vi "Build Update.vi"(8 "error in (no error)":errorcluster, 9 "tableName":string, 10 "DynamicParameters in":refnum<class "DynamicParameters.lvclass">, 11 "KDBConnection in":refnum<class "DBC.lvclass">) -> (0 "error out":errorcluster, 2 "Query":string, 3 "KDBConnection out":refnum<class "DBC.lvclass">)   [LabVIEW 2020, in "ORM_DBC_Kdb.lvlib" / "DBC.lvclass"]
uses:
  DBC.lvclass
  C:/Program Files/National Instruments/LabVIEW 2020/vi.lib/Viviota/shared/ORM.lvlibp/ORM/DbConnection/DbConnection.lvclass
  <vilib>/Viviota/shared/ORM.lvlibp/ORM/DynamicParameters/DynamicParameters.lvclass
  <vilib>/Viviota/shared/ORM.lvlibp/ORM/DbConnection/Read ColumnNameEqualsValueFormat.vi
  <vilib>/Viviota/shared/ORM.lvlibp/ORM/DbConnection/Write ExecuteScalar.vi
  <vilib>/Viviota/shared/ORM.lvlibp/ORM/DynamicParameters/Read FieldNames.vi
  <vilib>/Viviota/shared/ORM.lvlibp/ORM/DynamicParameters/Read ParameterNames.vi
  <vilib>/Viviota/shared/ORM.lvlibp/ORM/DynamicParameters/Read KeyProperties.vi
  <vilib>/Viviota/shared/ORM.lvlibp/ORM/DynamicParameters/Read AutoKey.vi
  <vilib>/Viviota/shared/ORM.lvlibp/ORM/DynamicParameters/Read ParameterOptions.vi
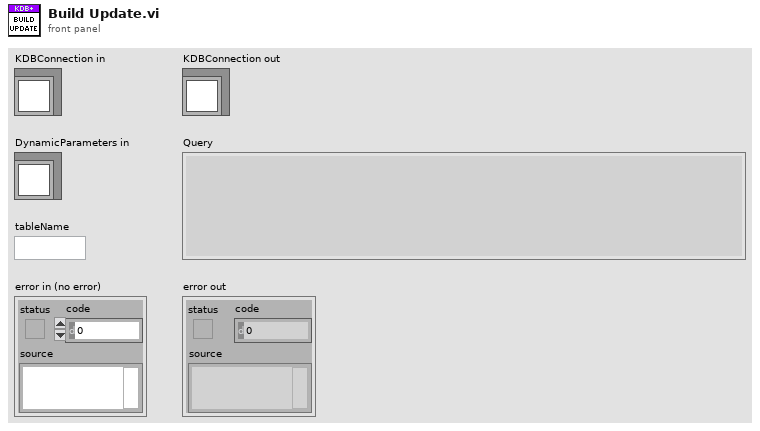
[diagram p1: front panel]
types:
  T1 = cluster{"DbType":i32, "Direction":i32, "Size":i32, "Precision":u8, "Scale":u8}[]
  T2 = typedef "ORM_DBC_Kdb.lvlib/DBC.lvclass/kdb_TableType_enum.ctl" = enum16{"Memory", "Disk_Serialized", "Disk_Splayed", "Disk_Partitioned", "Other"}
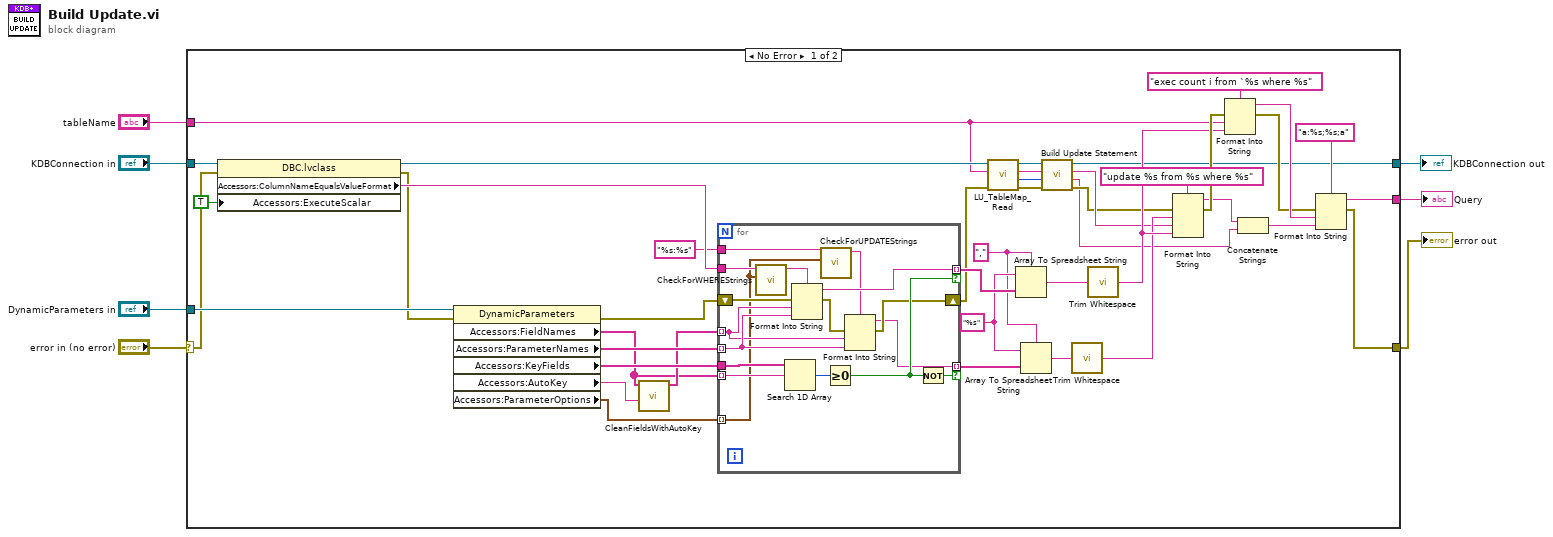
[diagram p0: block diagram]
diagram:
  n1 = case shown="No Error" "error in (no error)" {
    selector: "error in (no error)" -> [w45 w69]
    tunnel: [w28 w69] -> w2
    tunnel: [w13 w68] -> w6
    tunnel: "KDBConnection in" -> [w50 w68]
    tunnel: "DynamicParameters in" -> [w49 _]
    tunnel: "tableName" -> [w19 _]
    tunnel: [w33 _] -> w1
    frame No Error {
      w39 = "," ("delimiter (Tab)")
      w40 = "%s" ("format string")
      n2 = property class="DBC.lvclass"(reference=w50, error in=w45, "Accessors:ExecuteScalar"=TRUE ("ExecuteScalar")) -> (reference out=w20:refnum<class "DBC.lvclass">, error out=w44:errorcluster, "Accessors:ColumnNameEqualsValueFormat"=w47:string)
      n3 = property class="DynamicParameters"(reference=w49, error in=w44) -> (error out=w43:errorcluster, "Accessors:FieldNames"=w22:string[], "Accessors:ParameterNames"=w48:string[], "Accessors:KeyFields"=w42:string[], "Accessors:AutoKey"=w24:string, "Accessors:ParameterOptions"=w21:T1)  [unwired: 1 out]
      n4 = call "CleanFieldsWithAutoKey.vi"("AutoKey"=w24, "FieldNames"=w22) -> ("FieldNames_Clean"=w23:string[])  [unwired: 8 in, 1 out]
      n5 = for {
        tunnel: w23 -> [w61] mode=indexing
        tunnel: w48 -> [w62] mode=indexing
        tunnel: w47 -> [w55]
        tunnel: [w64] -> w46 mode=indexing if=w63
        shift-right: [w59] -> w18
        shift-left: w43 -> [w67]
        tunnel: w42 -> [w66]
        tunnel: [w58] -> w41 mode=indexing if=w57
        tunnel: "%s:%s" ("format string") -> [w52]
        tunnel: w22 -> [w56] mode=indexing
        tunnel: w21 -> [w51] mode=indexing
        n6 = call "CheckForWHEREStrings.vi"("Options"=w51, "ColumnNameEqualsValueFormat in"=w55) -> ("ColumnNameEqualsValueFormat out"=w54:string)  [unwired: 9 in]
        n7 = Search 1D Array(1D array=w66, element=w56) -> (index of element=w65:i32)  [unwired: 1 in]
        n8 = Format Into String(format string=w54, error in=w67, w61, w62) -> (resulting string=w64:string, error out=w60:errorcluster)  [unwired: 1 in]
        n9 = call "CheckForUPDATEStrings.vi"("Options"=w51, "DefaultFormat in"=w52) -> ("ActualFormat out"=w53:string)  [unwired: 9 in]
        n10 = Greater Or Equal To 0?(x=w65) -> (x >= 0?=w63:bool)
        n11 = Format Into String(format string=w53, error in=w60, w61, w62) -> (resulting string=w58:string, error out=w59:errorcluster)  [unwired: 1 in]
        n12 = Not(x=w63) -> (.not. x?=w57:bool)
      }
      n13 = call "LU_TableMap_Read.vi"("error in (no error)"=w18, "TableName"=w19, "KDBConnection in"=w20) -> ("error out"=w16:errorcluster, "TableType"=w14:T2, "TableName Out"=w15:string, "KDBConnection out"=w17:refnum<class "DBC.lvclass">)  [unwired: 5 in]
      n14 = Array To Spreadsheet String(delimiter (Tab)=w39, array=w46, 3:w40) -> (spreadsheet string=w37:string)
      n15 = Array To Spreadsheet String(delimiter (Tab)=w39, array=w41, 3:w40) -> (spreadsheet string=w34:string)
      n16 = call "Build Update Statement.vi"("error in (no error)"=w16, "TableType"=w14, "TableName Out"=w15, "KDBConnection in"=w17) -> ("error out"=w11:errorcluster, "Update Suffix Command"=w9:string, "Table to Use"=w12:string, "KDBConnection out"=w13:refnum<class "DBC.lvclass">)  [unwired: 4 in]
      n17 = call <vilib>:"Trim Whitespace.vi"("string"=w34) -> ("trimmed string"=w25:string)  [unwired: 1 in]
      n18 = call <vilib>:"Trim Whitespace.vi"("string"=w37) -> ("trimmed string"=w26:string)  [unwired: 1 in]
      n19 = Format Into String(format string="update %s from %s where %s", error in=w11, w25, w12, w26) -> (resulting string=w10:string, error out=w30:errorcluster)  [unwired: 1 in]
      n20 = Format Into String(format string="exec count i from `%s where %s", error in=w30, w19, w26) -> (resulting string=w31:string, error out=w29:errorcluster)  [unwired: 1 in]
      n21 = Concatenate Strings(w10, w9) -> (w8:string)
      n22 = Format Into String(format string="a:%s;%s;a", error in=w29, w31, w8) -> (resulting string=w33:string, error out=w28:errorcluster)  [unwired: 1 in]
    }
    frame Error {
    }
  }
  "error out" <- w2
  "KDBConnection out" <- w6
  "Query" <- w1
